vi "LVCAM Destroy Self.vi"(11 "Process in":refnum<class "ABD.lvclass">) -> (0 "error out":errorcluster, 1 "Destroyed Self?":bool, 3 "Process out":refnum<class "ABD.lvclass">)   [LabVIEW 2021, in "ABD.lvlib" / "ABD.lvclass"]
uses:
  ABD.lvclass
  ABD.lvclass/ABD.ctl
  LVCAM/LVCAM/LVCAM/LVCAM.lvclass
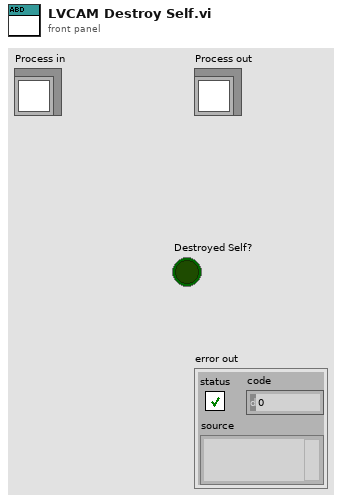
[diagram p1: front panel]
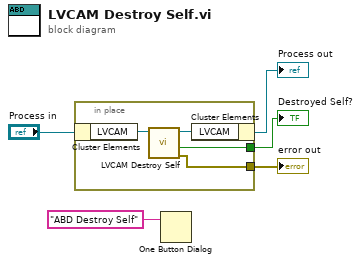
[diagram p0: block diagram]
diagram:
  n1 = in-place {
    in-place-border: [w7] -> w4
    in-place-border: [w6] -> w5
    n2 = in-place-cluster #1("Process in") -> ("LVCAM"=w9:refnum<class "LVCAM.lvclass">)
    n3 = call-dynamic "LVCAM Destroy Self.vi"("LVCAM Destroy Self in"=w9) -> ("error out"=w6:errorcluster, "Destroyed?"=w7:bool, "LVCAM Destroy Self out"=w8:refnum<class "LVCAM.lvclass">)  [unwired: 8 in]
    n4 = in-place-cluster #1("LVCAM"=w8) -> (→"Process out":refnum<class "ABD.lvclass">)
  }
  "error out" <- w5
  "Destroyed Self?" <- w4
  n5 = One Button Dialog(message="ABD Destroy Self") -> ()  [unwired: 1 in, 1 out]
